vi "FIU card.vi"(8 "error in (no error)":errorcluster, 11 "Node Ptr":T5 format="%.0x") -> (0 "error out":errorcluster)   [LabVIEW 2014, in "SLSC configuration System Explorer.lvlib"]
uses:
  SLSC configuration System Explorer.lvlib
  <vilib>/NI Veristand/Custom Device API/Custom Device Item Ref.ctl
  Type Defs/Card Position.ctl
  Shared/SPI Utility/Slot #.ctl
  Shared/FIU Board/Bank Fault States.ctl
  Shared/FIU Board/Fault State.ctl
  Shared/Constants.vi
  <vilib>/NI Veristand/Custom Device API/Get Item Property (U16).vi
  <vilib>/NI Veristand/Custom Device API/Custom Device API.lvlib
  Shared/SLSC configuration Shared.lvlib
panel:
  in  "Bank Fault States 1":T1
  in  "Header 3":cluster{"Section Name":string}={"Section Name"="Bank 1 Settings"}
  in  "Header 2":cluster{"Section Name":string}={"Section Name"="Bank 0 Settings"}
  in  "Bank Fault States 0":T1
  in  "Card Position":T3 {"Slot #" max=15}
  in  "Header":cluster{"Section Name":string}={"Section Name"="FIU Card Settings"}
  in  "Description":string
  in  "Name":string
  # "Fault 1"
  # "Fault 2"
  # "Fault 3"
  # "Fault 4"
  # "Fault 5"
  # "Fault 6"
  # "Fault 7"
  # "Fault 8"
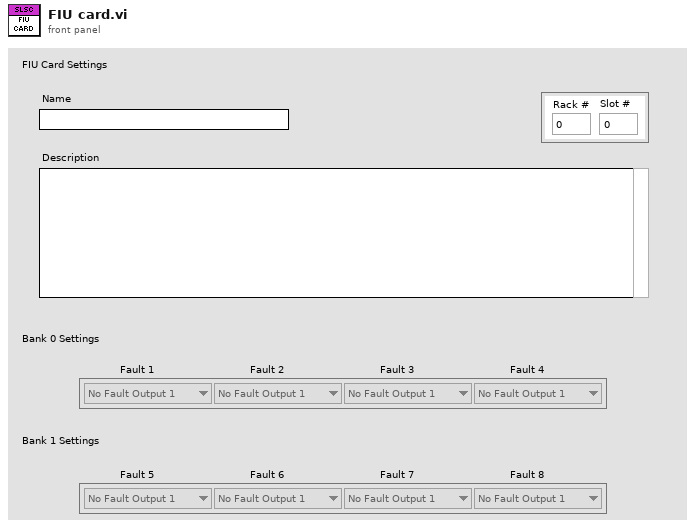
[diagram p1: front panel]
types:
  T1 = typedef "SLSC configuration Shared.lvlib/Bank Fault States.ctl" = T2[]
  T2 = typedef "SLSC configuration Shared.lvlib/Fault State.ctl" = enum8{"No Fault Output 1", "Open Circuit 100 Hz", "Ground 100 Hz", "Open Circuit", "Ground", "Fail Rail 1", "Fail Rail 2", "No Fault Output 2"}
  T3 = typedef "SLSC configuration Shared.lvlib/Card Position.ctl" = cluster{"Rack #":u8, "Slot #":T4}
  T4 = typedef "SLSC configuration Shared.lvlib/Slot #.ctl" = u8
  T5 = typedef "Custom Device API.lvlib/Custom Device Item Ref.ctl" = u64
  T6 = typedef "Custom Device API.lvlib/Custom Device Commands.ctl" = enum16{"Default", "Item renamed", "Shutdown", "Dynamic button pressed"}
  T7 = typedef "Custom Device API.lvlib/Custom Device Item Info.ctl" = cluster{"Name":string, "Is Channel":bool, "GUID":string, "Is Waveform":bool}
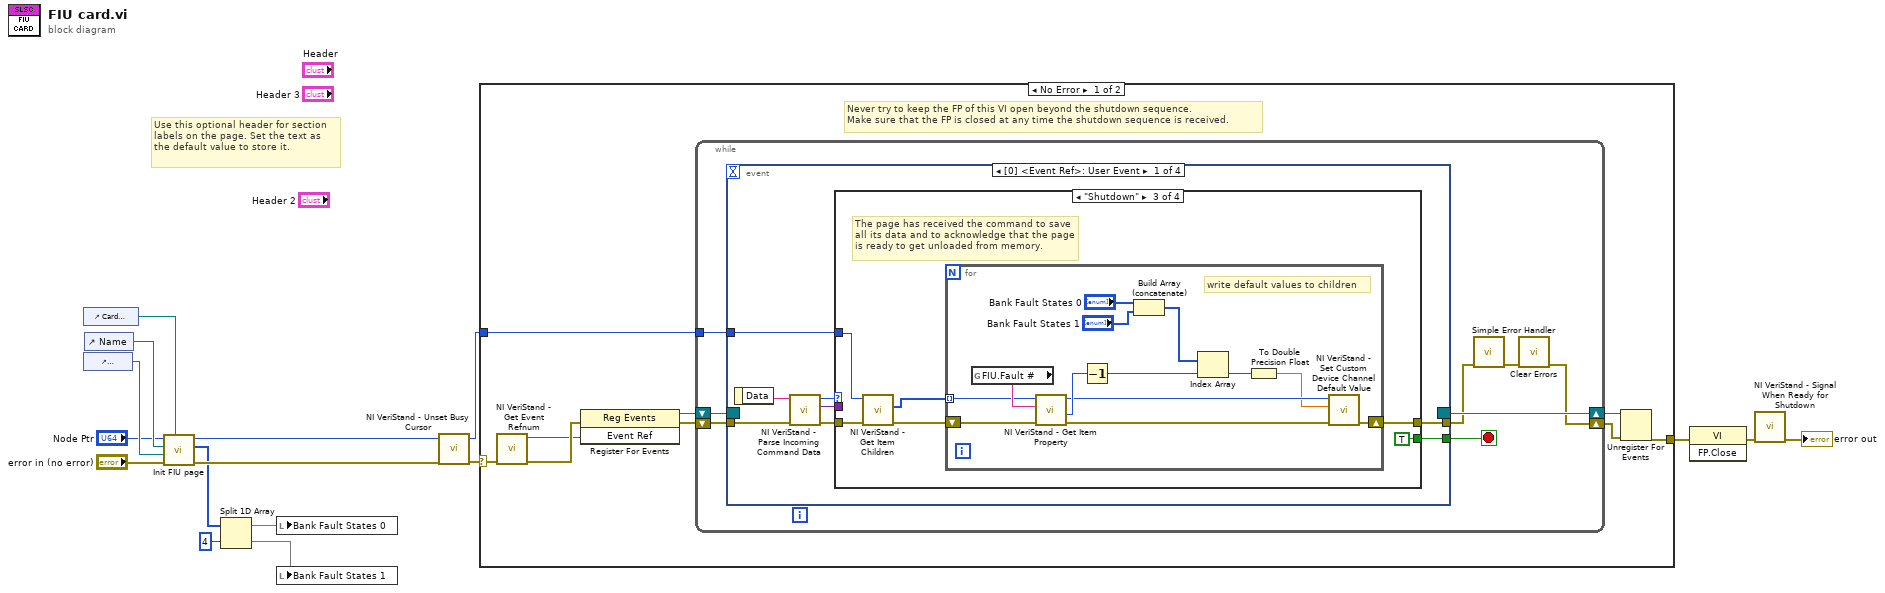
[diagram p0: block diagram]
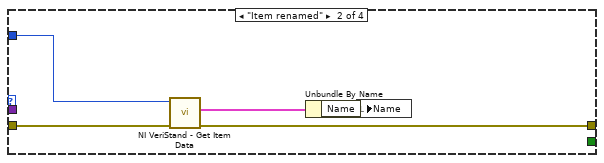
[diagram p3: hidden frame]
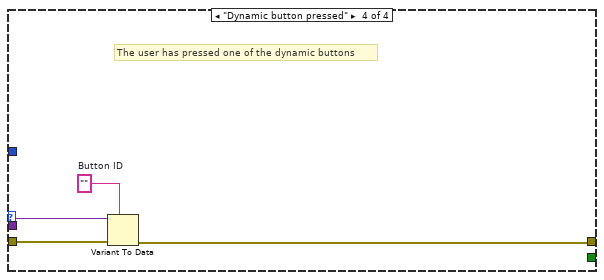
[diagram p4: hidden frame]
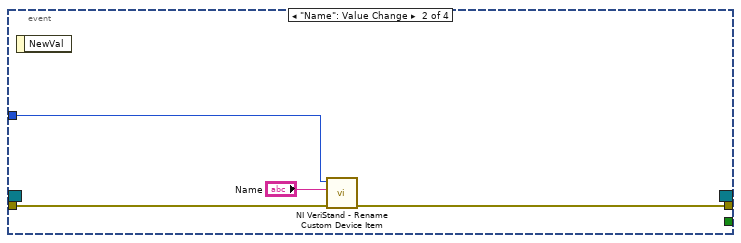
[diagram p5: hidden frame]
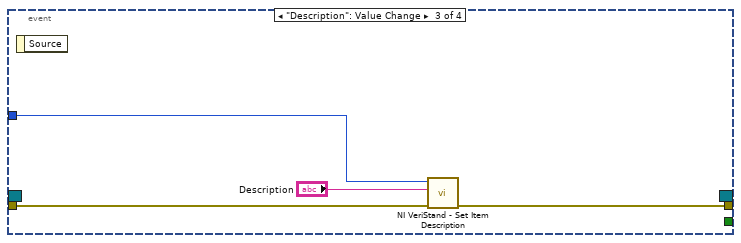
[diagram p6: hidden frame]
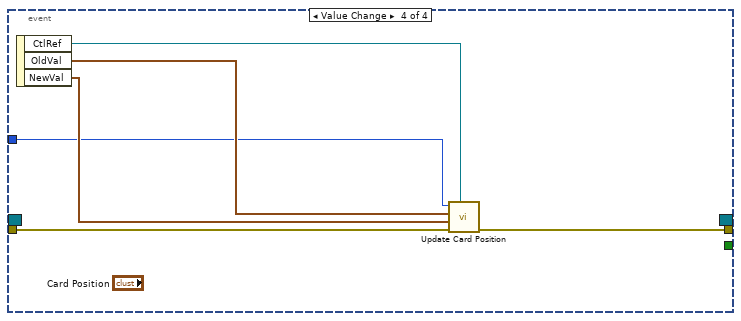
[diagram p7: hidden frame]
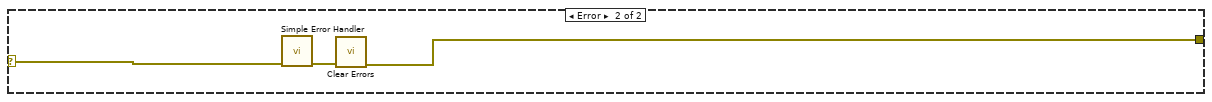
[diagram p8: hidden frame]
diagram:
  # "Use this optional header for section labels on the page. Set the text as the default value to store it."
  n1 = control-ref of="Card Position"() -> (w5:refnum<vi>)
  n2 = control-ref of="Description"() -> (w7:refnum<vi>)
  n3 = control-ref of="Name"() -> (w8:refnum<vi>)
  n4 = call "Init FIU page.vi"("Card Position"=w5, "error in (no error)"="error in (no error)", "Description"=w7, "Name"=w8, "Node Ptr"="Node Ptr") -> ("error out"=w12:errorcluster, "Fault States"=w4:T2[], "Node Ptr out"=w9:T5)  [unwired: 4 in]
  n5 = Split 1D Array(array=w4, index=4) -> (first subarray=w2:T2[], second subarray=w1:T2[])
  n6 = local write "Bank Fault States 0"(w2) -> ()
  n7 = local write "Bank Fault States 1"(w1) -> ()
  n8 = call <vilib>:"NI VeriStand - Unset Busy Cursor.vi"("error in (no error)"=w12) -> ("error out"=w11:errorcluster)  [unwired: 10 out]
  n9 = case shown="No Error" w11 {
    selector: w11 -> [w16 w86]
    tunnel: [w21 w84] -> w15
    tunnel: w9 -> [w17 _]
    frame No Error {
      # "Never try to keep the FP of this VI open beyond the shutdown sequence.\nMake sure that the FP is closed at any time the shutdown sequence is received."
      n10 = call <vilib>:"NI VeriStand - Get Event Refnum.vi"("error in (no error)"=w16) -> ("error out"=w24:errorcluster, "Event Ref"=w20:refnum<user-event>)  [unwired: 9 out]
      n11 = register-events(error in=w24, w20) -> (reference out=w18:refnum<event-registration>, error out=w19:errorcluster)  [unwired: 1 in]
      n12 = while {
        tunnel: w17 -> [w28]
        shift-right: [w25] -> w22
        shift-left: w19 -> [w31]
        shift-right: [w32] -> w23
        shift-left: w18 -> [w30]
        stop <- w29 stop-if-true
        n13 = event shown="[0] <Event Ref>: User Event" {
          selector: w30 -> [_ _ _ _]
          dyn-events: [_ _ _ _] -> w32
          timeout: _ -> [_ _ _ _]
          tunnel: w31 -> [w40 w73 w76 w82]
          tunnel: [w36 _ _ _] -> w29
          tunnel: [w35 w72 w75 w83] -> w27
          tunnel: w28 -> [w34 w71 w77 w79]
          event User Event {
            n14 = event-data() -> ("Data"=w39:string)  [unwired: 1 out]
            n15 = call <vilib>:"NI VeriStand - Parse Incoming Command Data.vi"("error in (no error)"=w40, "Incoming data"=w39) -> ("error out"=w38:errorcluster, "Outgoing data"=w33:variant, "Action"=w37:T6)  [unwired: 7 out]
            n16 = case shown="\"Shutdown\"" w37 {
              tunnel: w38 -> [w41 w46 w49 w69]
              tunnel: [_ _ TRUE _] -> w36
              tunnel: [w41 w43 w51 w66] -> w35
              tunnel: w34 -> [_ w45 w47 _]
              tunnel: w33 -> [_ _ _ w68]
              frame "Default", Default {
              }
              frame "Item renamed" {
                n17 = call <vilib>:"NI VeriStand - Get Item Data.vi"("error in (no error)"=w46, "Item Ref in"=w45) -> ("error out"=w43:errorcluster, "Item Info"=w44:T7)  [unwired: 8 out]
                n18 = Unbundle By Name(w44) -> ("Name"=w42:string)
                n19 = local write "Name"(w42) -> ()
              }
              frame "Shutdown" {
                # "The page has received the command to save all its data and to acknowledge that the page is ready to get unloaded from memory."
                n20 = call <vilib>:"NI VeriStand - Get Item Children.vi"("error in (no error)"=w49, "Item Ref in"=w47) -> ("error out"=w48:errorcluster, "Child Refs"=w50:T5[])  [unwired: 6 in, 2 out]
                n21 = for {
                  shift-right: [w62] -> w51
                  shift-left: w48 -> [w64]
                  tunnel: w50 -> [w59] mode=indexing
                  # "write default values to children"
                  n22 = global read "Constants.vi" "FIU.Fault #"() -> (w65:string)
                  n23 = call-poly <vilib>:"NI VeriStand - Get Item Property.vi"("error in (no error)"=w64, "Property Name"=w65, "Item Ref in"=w59) -> ("error out"=w53:errorcluster, "Value"=w63:u16, "Item Ref out"=w61:T5)  [unwired: 5 in, 1 out]
                  n24 = Decrement(x=w63) -> (x-1=w55:u16)
                  n25 = Build Array (concatenate)("Bank Fault States 0", "Bank Fault States 1") -> (w56:T1)
                  n26 = Index Array(array=w56, index=w55) -> (element=w54:T2)
                  n27 = To Double Precision Float(number=w54) -> (double precision float=w60:dbl)
                  n28 = call <vilib>:"NI VeriStand - Set Custom Device Channel Default Value.vi"("error in (no error)"=w53, "Default Value"=w60, "Channel Ref in"=w61) -> ("error out"=w62:errorcluster)  [unwired: 7 in, 1 out]
                }
              }
              frame "Dynamic button pressed" {
                w67 = ""  # Button ID
                # "The user has pressed one of the dynamic buttons"
                n29 = Variant To Data(error in=w69, type=w67, Variant=w68) -> (error out=w66:errorcluster)  [unwired: 1 out]
              }
            }
          }
          event "Name": Value Change {
            n30 = event-data() -> ()  [unwired: 2 out]
            n31 = call <vilib>:"NI VeriStand - Rename Custom Device Item.vi"("error in (no error)"=w73, "New Name"="Name", "Item Ref in"=w71) -> ("error out"=w72:errorcluster)  [unwired: 1 in, 7 out]
          }
          event "Description": Value Change {
            n32 = event-data() -> ()  [unwired: 2 out]
            n33 = call <vilib>:"NI VeriStand - Set Item Description.vi"("error in (no error)"=w76, "Description"="Description", "Item Ref in"=w77) -> ("error out"=w75:errorcluster)  [unwired: 8 out]
          }
          event Value Change {
            n34 = event-data() -> ("CtlRef"=w78:refnum<vi>, "OldVal"=w80:T3, "NewVal"=w81:T3)  [unwired: 1 out]
            n35 = call "Update Card Position.vi"("Card Position Ref"=w78, "error in (no error)"=w82, "NewVal"=w81, "OldVal"=w80, "Node Ptr in"=w79) -> ("error out"=w83:errorcluster)  [unwired: 6 in]
          }
        }
        n36 = call <vilib>:"Simple Error Handler.vi"("error in (no error)"=w27) -> ("error out"=w26:errorcluster)  [unwired: 1 in, 7 out]
        n37 = call <vilib>:"Clear Errors.vi"("error in (no error)"=w26) -> ("error out"=w25:errorcluster)  [unwired: 1 in, 5 out]
      }
      n38 = Unregister For Events(event registration refnum=w23, error in=w22) -> (error out=w21:errorcluster)
    }
    frame Error {
      n39 = call <vilib>:"Simple Error Handler.vi"("error in (no error)"=w86) -> ("error out"=w85:errorcluster)  [unwired: 1 in, 7 out]
      n40 = call <vilib>:"Clear Errors.vi"("error in (no error)"=w85) -> ("error out"=w84:errorcluster)  [unwired: 1 in, 5 out]
    }
  }
  n41 = invoke class="VI" method="FP.Close"(error in=w15) -> (error out=w14:errorcluster)  [unwired: 2 in, 2 out]
  n42 = call <vilib>:"NI VeriStand - Signal When Ready for Shutdown.vi"("error in (no error)"=w14) -> ("error out"=→"error out":errorcluster)  [unwired: 10 out]
